vi "Block Test.vi"() -> ()   [LabVIEW 2016]
uses:
  Source/GE 5565PIORC/Controls/Interrupt Enables.ctl
  Source/GE 5565PIORC/GE 5565PIORC.lvclass/GE 5565PIORC.ctl
  Source/GE 5565PIORC/Controls/DMA Transfer Spec (Block).ctl
  Source/GE 5565PIORC/Controls/DMA Block Descriptor.ctl
  Source/GE 5565PIORC/VIs/Binary Operations/Set Bits.vi
  Source/GE 5565PIORC/VIs/Binary Operations/Set Bits U32.vi
  Source/GE 5565PIORC/VIs/Registers/Local Configuration.Get Register Offset.vi
  Source/GE 5565PIORC/VIs/Binary Operations/Get Bits.vi
  Source/GE 5565PIORC/VIs/Binary Operations/Get Bits U32.vi
  Source/GE 5565PIORC/VIs/Registers/RFM Control and Status.Get Register Offset.vi
  Source/GE 5565PIORC/VIs/DMA/DMA.Configure.vi
  Source/GE 5565PIORC/VIs/DMA/DMA.Configure (Block).vi
  Source/GE 5565PIORC/VIs/Registers/Local Configuration.DMAMODE0.Scatter-Gather Enable.Set.vi
  Source/GE 5565PIORC/VIs/Registers/Local Configuration.PCI Address.Set.vi
  Source/GE 5565PIORC/VIs/Registers/Local Configuration.Local Address.Set.vi
  Source/GE 5565PIORC/VIs/Registers/Local Configuration.Transfer Size.Set.vi
  Source/GE 5565PIORC/VIs/Registers/Local Configuration.DMADPR0.Transfer Direction.Set.vi
  Source/GE 5565PIORC/VIs/Registers/Local Configuration.DMACSR0.DMA Start.Set.vi
  Source/GE 5565PIORC/VIs/Registers/Local Configuration.DMACSR0.DMA Clear Interrupt.Set.vi
  <vilib>/Utility/error.llb/Clear Errors.vi
  Source/GE 5565PIORC/GE 5565PIORC.lvclass
  <instrlib>/GE 5565 PIORC/GE 5565 PIORC.lvlib
panel:
  out "Delayed Read Mode Enabled?":bool
  out "Timed out? 2":bool
  out "Data out":dbl[](array[numeric])
  out "us period 2":u32
  out "us read period":u32
  in  "value":dbl
  in  "index":i32
  out "Data in":dbl[](array[numeric])
  out "Timed out?":bool
  in  "timeout ms (1000)":u32=1000
  out "us period":u32
  in  "data size":i32=10000
  in  "stop":bool
  in  "RFM Address":u32 format="%08x"
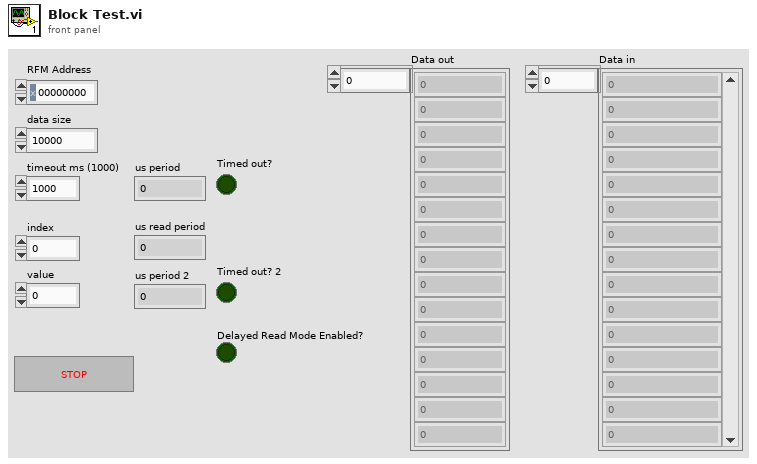
[diagram p1: front panel]
types:
  T1 = typedef "GE 5565PIORC.lvclass/Interrupt Enables.ctl" = cluster{"PCI Interrupt":bool, "Local Interrupt":bool, "DMA Interrupt":bool}
  T2 = cluster{"VMIC 5565 Resource":refnum<visa-resource-name>, "MEMACC Resource":refnum<visa-resource-name>, "byte count":u32, "mem offset":u32}
  T3 = typedef "GE 5565PIORC.lvclass/DMA Block Descriptor.ctl" = cluster{"descriptor ptr (VISA)":u32, "descriptor size":u32, "descriptor ptr (aligned)":u32, "data ptr (lower)":u32, "data ptr (upper)":u32, "data size":u32, "next descriptor ptr":u32}
  T4 = typedef "GE 5565PIORC.lvclass/DMA Transfer Spec (Block).ctl" = cluster{"RFM Address":u32, "Block Descriptor":T3}
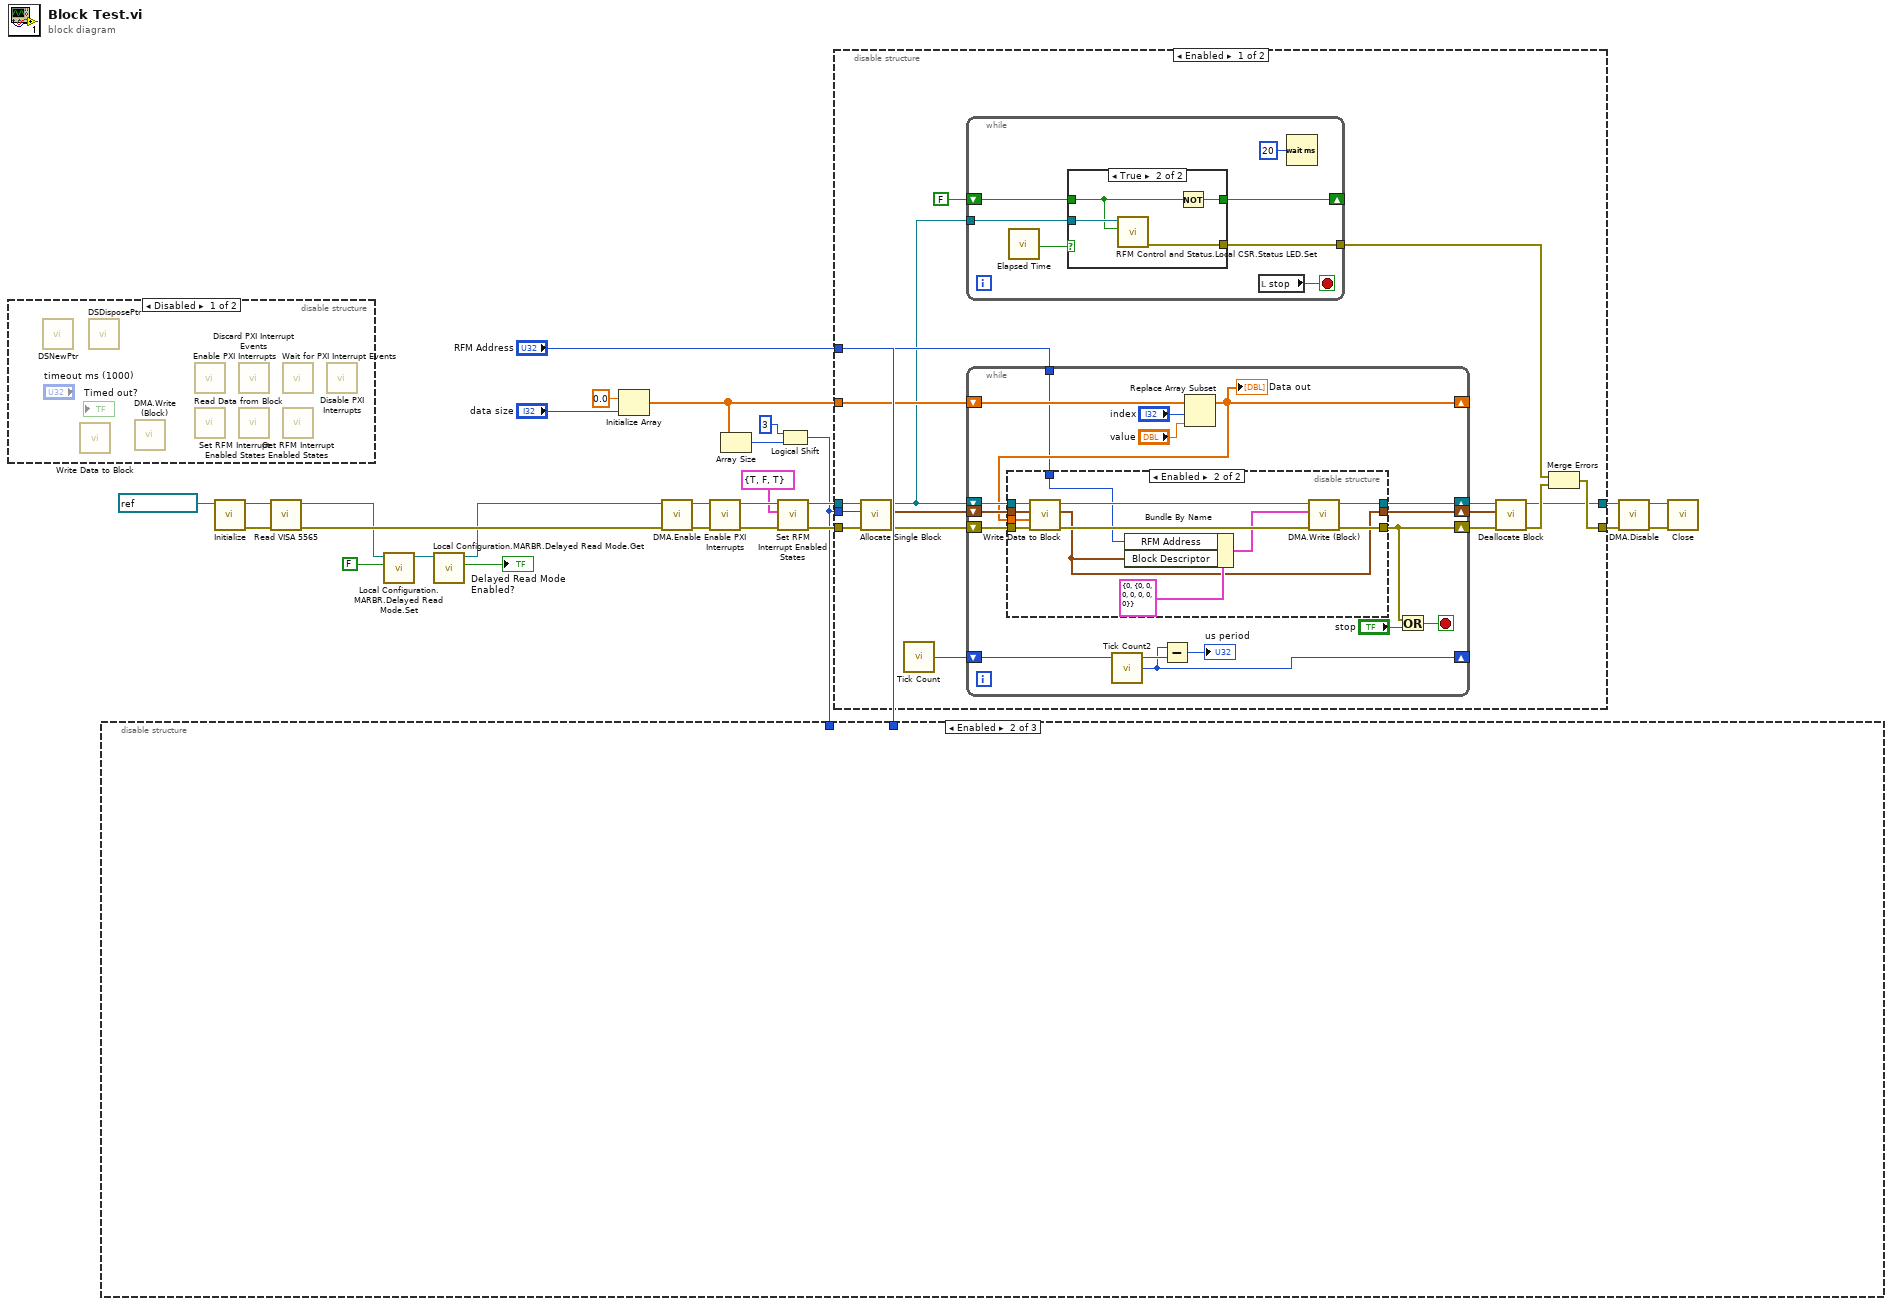
[diagram p0: block diagram]
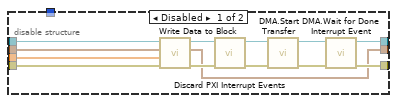
[diagram p3: hidden frame]
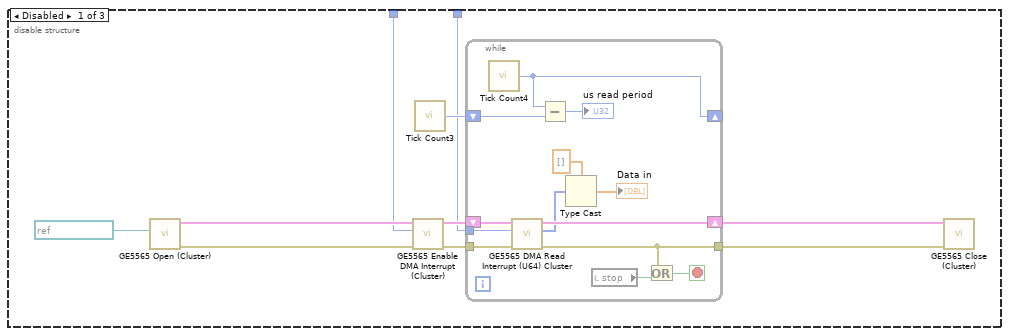
[diagram p5: hidden frame]
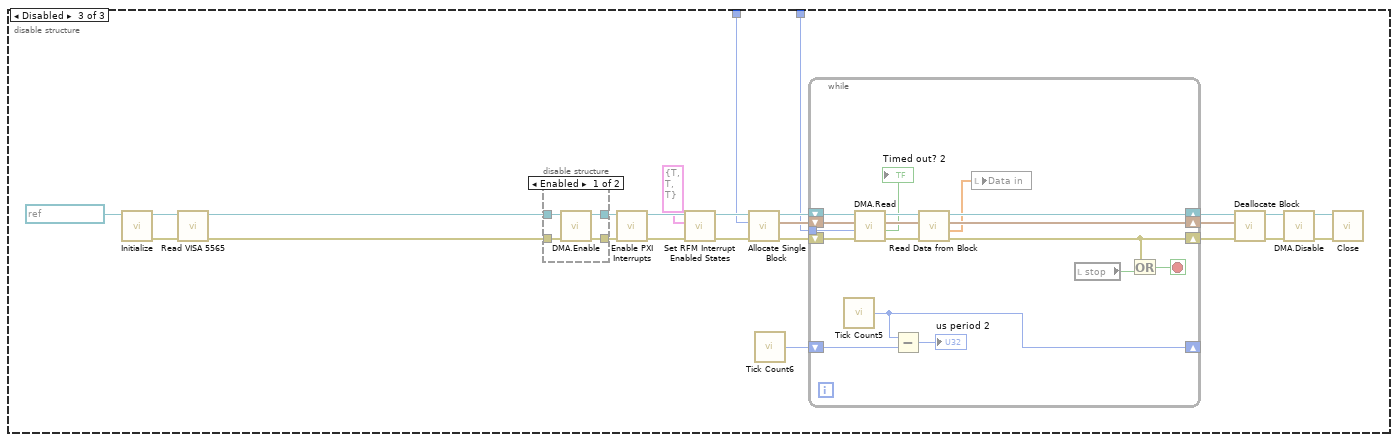
[diagram p6: hidden frame]
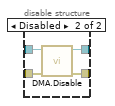
[diagram p7: hidden frame]
diagram:
  n1 = disable-structure shown="Disabled" {
    frame Disabled {
      n2 = call <vilib>:"DSNewPtr.vi"() -> ()  [unwired: 10 in, 2 out]
      n3 = call "Write Data to Block.vi"() -> ()  [unwired: 9 in, 3 out]
      n4 = call <vilib>:"DSDisposePtr.vi"() -> ()  [unwired: 11 in, 1 out]
      n5 = call "DMA.Write (Block).vi"() -> ()  [unwired: 9 in, 3 out]
      n6 = call "Enable PXI Interrupts.vi"() -> ()  [unwired: 10 in, 2 out]
      n7 = call "Read Data from Block.vi"() -> ()  [unwired: 8 in, 4 out]
      n8 = call "Discard PXI Interrupt Events.vi"() -> ()  [unwired: 10 in, 2 out]
      n9 = call "Set RFM Interrupt Enabled States.vi"() -> ()  [unwired: 10 in, 2 out]
      n10 = call "Wait for PXI Interrupt Events.vi"() -> ()  [unwired: 9 in, 3 out]
      n11 = call "Get RFM Interrupt Enabled States.vi"() -> ()  [unwired: 9 in, 3 out]
      n12 = call "Disable PXI Interrupts.vi"() -> ()  [unwired: 10 in, 2 out]
    }
    frame Enabled {
    }
  }
  n13 = call "Initialize.vi"("VISA resource name"=refnum<visa-resource-name> "RefMem2") -> ("error out"=w7:errorcluster, "GE 5565PIORC"=w8:refnum<class "GE 5565PIORC.lvclass">)  [unwired: 9 in]
  n14 = call "Read VISA 5565.vi"("error in (no error)"=w7, "GE 5565PIORC in"=w8) -> ("error out"=w6:errorcluster, "GE 5565PIORC out"=w2:refnum<class "GE 5565PIORC.lvclass">)  [unwired: 7 in, 1 out]
  n15 = call "Local Configuration.MARBR.Delayed Read Mode.Set.vi"("Enable Delayed Read Mode?"=FALSE, "GE 5565PIORC"=w2) -> ("GE 5565PIORC out"=w3:refnum<class "GE 5565PIORC.lvclass">)  [unwired: 8 in, 1 out]
  n16 = call "Local Configuration.MARBR.Delayed Read Mode.Get.vi"("GE 5565PIORC"=w3) -> ("Delayed Read Mode Enabled?"=→"Delayed Read Mode Enabled?":bool, "GE 5565PIORC out"=w5:refnum<class "GE 5565PIORC.lvclass">)  [unwired: 8 in, 1 out]
  n17 = Initialize Array(0.0 ("element"), "data size") -> (w15:dbl[])
  n18 = call "DMA.Enable.vi"("error in (no error)"=w6, "GE 5565PIORC in"=w5) -> ("error out"=w23:errorcluster, "GE 5565PIORC out"=w24:refnum<class "GE 5565PIORC.lvclass">)  [unwired: 8 in]
  n19 = call "Enable PXI Interrupts.vi"("error in (no error)"=w23, "GE 5565PIORC in"=w24) -> ("error out"=w21:errorcluster, "GE 5565PIORC out"=w22:refnum<class "GE 5565PIORC.lvclass">)  [unwired: 8 in]
  n20 = Array Size(array=w15) -> (size(s)=w26:i32)
  n21 = call "Set RFM Interrupt Enabled States.vi"("error in (no error)"=w21, "Interrupt Enables"=T1 {"PCI Interrupt"=TRUE, "Local Interrupt"=FALSE, "DMA Interrupt"=TRUE}, "GE 5565PIORC in"=w22) -> ("error out"=w19:errorcluster, "GE 5565PIORC out"=w20:refnum<class "GE 5565PIORC.lvclass">)  [unwired: 7 in]
  n22 = Logical Shift(y=i16 3, x=w26) -> (x << y=w10:i32)
  n23 = disable-structure shown="Enabled" {
    disable-tunnel: w10 -> [w34 _ w56]
    disable-tunnel: "RFM Address" -> [w28 _ w55]
    frame Disabled {
      n24 = call <instrlib>:"GE5565 Open (Cluster).vi"("VISA resource name (empty)"=refnum<visa-resource-name> "RefMem1") -> ("error out"=w35:errorcluster, "VMIC-5565"=w36:T2)  [unwired: 5 in]
      n25 = call <instrlib>:"GE5565 Enable DMA Interrupt (Cluster).vi"("error in (no error)"=w35, "transfer size (1024 bytes)"=w34, "VMIC reference in"=w36) -> ("error out"=w32:errorcluster, "VMIC reference out"=w33:T2)  [unwired: 3 in]
      n26 = call "Tick Count3"() -> ("Tick Count(uSec)"=w29:u32)
      n27 = while {
        tunnel: w32 -> [w41]
        shift-right: [w42] -> w31
        shift-left: w33 -> [w43]
        tunnel: [w40] -> w30
        shift-right: [w46] -> _
        shift-left: w29 -> [w45]
        tunnel: w28 -> [w38]
        stop <- w47 stop-if-true
        n28 = call "Tick Count4"() -> ("Tick Count(uSec)"=w46:u32)
        n29 = call "GE5565 DMA Read Interrupt (U64) Cluster.vi"("error in (no error)"=w41, "offset (0)"=w38, "VMIC reference in"=w43) -> ("error out"=w40:errorcluster, "buffer"=w39:u64[], "VMIC reference out"=w42:T2)  [unwired: 6 in]
        n30 = Subtract(x=w46, y=w45) -> (x-y=→"us read period":u32)
        n31 = Type Cast(type=dbl[] [], x=w39) -> (*(type *) &x=→"Data in":dbl[])
        n32 = local read "stop"() -> (w48:bool)
        n33 = Or(x=w40, y=w48) -> (x .or. y?=w47:bool)
      }
      n34 = call <instrlib>:"GE5565 Close (Cluster).vi"("error in (no error)"=w30, "VMIC reference in"=w31) -> ()  [unwired: 5 in, 1 out]
    }
    frame Enabled {
    }
    frame Disabled {
      n35 = call "Initialize.vi"("VISA resource name"=refnum<visa-resource-name> "RefMem1") -> ("error out"=w52:errorcluster, "GE 5565PIORC"=w54:refnum<class "GE 5565PIORC.lvclass">)  [unwired: 9 in]
      n36 = call "Read VISA 5565.vi"("error in (no error)"=w52, "GE 5565PIORC in"=w54) -> ("error out"=w51:errorcluster, "GE 5565PIORC out"=w53:refnum<class "GE 5565PIORC.lvclass">)  [unwired: 7 in, 1 out]
      n37 = disable-structure shown="Enabled" {
        disable-tunnel: w51 -> [w79 w82]
        disable-tunnel: [w78 w81] -> w74
        disable-tunnel: [w77 w80] -> w73
        disable-tunnel: w53 -> [w76 w83]
        frame Enabled {
          n38 = call "DMA.Enable.vi"("error in (no error)"=w79, "GE 5565PIORC in"=w76) -> ("error out"=w77:errorcluster, "GE 5565PIORC out"=w78:refnum<class "GE 5565PIORC.lvclass">)  [unwired: 8 in]
        }
        frame Disabled {
          n39 = call "DMA.Disable.vi"("error in (no error)"=w82, "GE 5565PIORC in"=w83) -> ("error out"=w80:errorcluster, "GE 5565PIORC out"=w81:refnum<class "GE 5565PIORC.lvclass">)  [unwired: 8 in]
        }
      }
      n40 = call "Enable PXI Interrupts.vi"("error in (no error)"=w73, "GE 5565PIORC in"=w74) -> ("error out"=w71:errorcluster, "GE 5565PIORC out"=w72:refnum<class "GE 5565PIORC.lvclass">)  [unwired: 8 in]
      n41 = call "Set RFM Interrupt Enabled States.vi"("error in (no error)"=w71, "Interrupt Enables"=T1 {"PCI Interrupt"=TRUE, "Local Interrupt"=TRUE, "DMA Interrupt"=TRUE}, "GE 5565PIORC in"=w72) -> ("error out"=w69:errorcluster, "GE 5565PIORC out"=w70:refnum<class "GE 5565PIORC.lvclass">)  [unwired: 7 in]
      n42 = call "Allocate Single Block.vi"("error in (no error)"=w69, "size (bytes)"=w56, "GE 5565PIORC in"=w70) -> ("error out"=w63:errorcluster, "Block Descriptor"=w62:T3, "GE 5565PIORC out"=w64:refnum<class "GE 5565PIORC.lvclass">)  [unwired: 6 in]
      n43 = call "Tick Count6"() -> ("Tick Count(uSec)"=w57:u32)
      n44 = while {
        shift-right: [w89] -> w67
        shift-left: w64 -> [w96]
        shift-right: [w87] -> w65
        shift-left: w63 -> [w95]
        shift-right: [w88] -> w66
        shift-left: w62 -> [w94]
        shift-right: [w97] -> _
        shift-left: w57 -> [w99]
        tunnel: w55 -> [w93]
        stop <- w100 stop-if-true
        n45 = call "Tick Count5"() -> ("Tick Count(uSec)"=w97:u32)
        n46 = call "DMA.Read.vi"("error in (no error)"=w95, "RFM Address"=w93, "Block Descriptor"=w94, "GE 5565PIORC"=w96) -> ("error out"=w92:errorcluster, "Timed out?"=→"Timed out? 2":bool, "Block Descriptor out"=w90:T3, "GE 5565PIORC out"=w91:refnum<class "GE 5565PIORC.lvclass">)  [unwired: 4 in]
        n47 = Subtract(x=w97, y=w99) -> (x-y=→"us period 2":u32)
        n48 = call "Read Data from Block.vi"("error in (no error)"=w92, "Block Descriptor"=w90, "GE 5565PIORC"=w91) -> ("error out"=w87:errorcluster, "Data"=w86:dbl[], "Block Descriptor out"=w88:T3, "GE 5565PIORC out"=w89:refnum<class "GE 5565PIORC.lvclass">)  [unwired: 5 in]
        n49 = local write "Data in"(w86) -> ()
        n50 = local read "stop"() -> (w85:bool)
        n51 = Or(x=w87, y=w85) -> (x .or. y?=w100:bool)
      }
      n52 = call "Deallocate Block.vi"("error in (no error)"=w65, "Block Descriptor"=w66, "GE 5565PIORC in"=w67) -> ("error out"=w60:errorcluster, "GE 5565PIORC out"=w61:refnum<class "GE 5565PIORC.lvclass">)  [unwired: 7 in]
      n53 = call "DMA.Disable.vi"("error in (no error)"=w60, "GE 5565PIORC in"=w61) -> ("error out"=w58:errorcluster, "GE 5565PIORC out"=w59:refnum<class "GE 5565PIORC.lvclass">)  [unwired: 8 in]
      n54 = call "Close.vi"("error in (no error)"=w58, "GE 5565PIORC in"=w59) -> ()  [unwired: 9 in, 1 out]
    }
  }
  n55 = disable-structure shown="Enabled" {
    disable-tunnel: w20 -> [w117 w172]
    disable-tunnel: w19 -> [w116 w171]
    disable-tunnel: w15 -> [w114 _]
    disable-tunnel: [w101 w172] -> w14
    disable-tunnel: [w103 w171] -> w13
    disable-tunnel: w10 -> [w110 _]
    disable-tunnel: "RFM Address" -> [w112 _]
    frame Enabled {
      n56 = call "Allocate Single Block.vi"("error in (no error)"=w116, "size (bytes)"=w110, "GE 5565PIORC in"=w117) -> ("error out"=w109:errorcluster, "Block Descriptor"=w111:T3, "GE 5565PIORC out"=w107:refnum<class "GE 5565PIORC.lvclass">)  [unwired: 6 in]
      n57 = call "Tick Count"() -> ("Tick Count(uSec)"=w113:u32)
      n58 = while {
        shift-right: [w119] -> _
        shift-left: FALSE -> [w122]
        tunnel: w107 -> [w121]
        tunnel: [w118] -> w102
        stop <- w120 stop-if-true
        n59 = call "Elapsed Time"() -> ("Time has Elapsed"=w123:bool)  [unwired: 12 in, 7 out]
        n60 = case shown="True" w123 {
          tunnel: w122 -> [w125 w127]
          tunnel: w121 -> [_ w129]
          tunnel: [w125 w128] -> w119
          tunnel: [_ w126] -> w118
          frame False {
          }
          frame True {
            n61 = call "RFM Control and Status.Local CSR.Status LED.Set.vi"("Status LED State"=w127, "GE 5565PIORC"=w129) -> ("error out"=w126:errorcluster)  [unwired: 8 in, 1 out]
            n62 = Not(x=w127) -> (.not. x?=w128:bool)
          }
        }
        n63 = local read "stop"() -> (w120:bool)
        n64 = Wait (ms)(milliseconds to wait=u32 20) -> ()  [unwired: 1 out]
      }
      n65 = while {
        tunnel: w112 -> [w130]
        shift-right: [w137] -> w115
        shift-left: w107 -> [w135]
        shift-right: [w136] -> w105
        shift-left: w109 -> [w134]
        shift-right: [w131] -> w106
        shift-left: w111 -> [w133]
        shift-right: [w132] -> _
        shift-left: w114 -> [w141]
        shift-right: [w140] -> _
        shift-left: w113 -> [w143]
        stop <- w144 stop-if-true
        n66 = call "Tick Count2"() -> ("Tick Count(uSec)"=w140:u32)
        n67 = Subtract(x=w140, y=w143) -> (x-y=→"us period":u32)
        n68 = Replace Array Subset(array=w141, new element="value", index="index") -> (w132:dbl[])
        "Data out" <- w132
        n69 = disable-structure shown="Enabled" {
          disable-tunnel: [w154 w164] -> w137
          disable-tunnel: [w153 w170] -> w136
          disable-tunnel: w135 -> [w151 w166]
          disable-tunnel: w134 -> [w149 w169]
          disable-tunnel: w133 -> [w148 w168]
          disable-tunnel: w132 -> [w147 w167]
          disable-tunnel: [w146 w161] -> w131
          disable-tunnel: w130 -> [_ w160]
          frame Disabled {
            n70 = call "Write Data to Block.vi"("error in (no error)"=w149, "Data"=w147, "Block Descriptor"=w148, "GE 5565PIORC"=w151) -> ("error out"=w150:errorcluster, "Block Descriptor out"=w146:T3, "GE 5565PIORC out"=w152:refnum<class "GE 5565PIORC.lvclass">)  [unwired: 5 in]
            n71 = call "Discard PXI Interrupt Events.vi"("error in (no error)"=w150, "GE 5565PIORC in"=w152) -> ("error out"=w158:errorcluster, "GE 5565PIORC out"=w156:refnum<class "GE 5565PIORC.lvclass">)  [unwired: 8 in]
            n72 = call "DMA.Start Transfer.vi"("error in (no error)"=w158, "GE 5565PIORC"=w156) -> ("error out"=w157:errorcluster, "GE 5565PIORC out"=w155:refnum<class "GE 5565PIORC.lvclass">)  [unwired: 8 in]
            n73 = call "DMA.Wait for Done Interrupt Event.vi"("error in (no error)"=w157, "GE 5565PIORC"=w155) -> ("error out"=w153:errorcluster, "GE 5565PIORC out"=w154:refnum<class "GE 5565PIORC.lvclass">)  [unwired: 7 in, 1 out]
          }
          frame Enabled {
            n74 = call "Write Data to Block.vi"("error in (no error)"=w169, "Data"=w167, "Block Descriptor"=w168, "GE 5565PIORC"=w166) -> ("error out"=w163:errorcluster, "Block Descriptor out"=w161:T3, "GE 5565PIORC out"=w165:refnum<class "GE 5565PIORC.lvclass">)  [unwired: 5 in]
            n75 = Bundle By Name(cluster=T4 {"RFM Address"=0, "Block Descriptor"={"descriptor ptr (VISA)"=0, "descriptor size"=0, "descriptor ptr (aligned)"=0, "data ptr (lower)"=0, "data ptr (upper)"=0, "data size"=0, "next descriptor ptr"=0}} ("Transfer Spec (Block)"), "RFM Address"=w160, "Block Descriptor"=w161) -> (w159:T4)
            n76 = call "DMA.Write (Block).vi"("error in (no error)"=w163, "Block Transfer Spec"=w159, "GE 5565PIORC"=w165) -> ("error out"=w170:errorcluster, "GE 5565PIORC out"=w164:refnum<class "GE 5565PIORC.lvclass">)  [unwired: 6 in, 1 out]
          }
        }
        n77 = Or(x=w136, y="stop") -> (x .or. y?=w144:bool)
      }
      n78 = call "Deallocate Block.vi"("error in (no error)"=w105, "Block Descriptor"=w106, "GE 5565PIORC in"=w115) -> ("error out"=w104:errorcluster, "GE 5565PIORC out"=w101:refnum<class "GE 5565PIORC.lvclass">)  [unwired: 7 in]
      n79 = Merge Errors(w102, w104) -> (w103:errorcluster)
    }
    frame Disabled {
    }
  }
  n80 = call "DMA.Disable.vi"("error in (no error)"=w13, "GE 5565PIORC in"=w14) -> ("error out"=w11:errorcluster, "GE 5565PIORC out"=w12:refnum<class "GE 5565PIORC.lvclass">)  [unwired: 8 in]
  n81 = call "Close.vi"("error in (no error)"=w11, "GE 5565PIORC in"=w12) -> ()  [unwired: 9 in, 1 out]
